vi "test_delay.vi"() -> ()   [LabVIEW 2013]
uses:
  <vilib>/rvi/FXPMathLib/FxpConvert/subVIs/nifxpmath_Convert_SimConfig.ctl
  <vilib>/fxp/LVFixedPointQuantizationPolicyTypeDef.ctl
  <vilib>/fxp/LVFixedPointOverflowPolicyTypeDef.ctl
  <vilib>/rvi/FXPMathLib/FxpConvert/simVIs/DllFxpConvertTemp_sub.vi
  <vilib>/rvi/FXPMathLib/FxpConvert/XNode/nifxpmath_Convert.xnode
  <vilib>/rvi/FXPMathLib/FxpMul/XNode/nifxpmath_Multiplier.xnode
  <vilib>/rvi/FXPMathLib/sim/FxpSim.dll
panel:
  out "Array 2":fxp<+/-,32,16>[](array[numeric])
  out "Array":fxp<+/-,16,14>[](array[numeric])
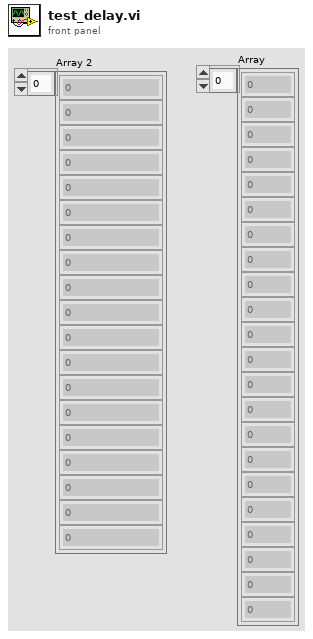
[diagram p1: front panel]
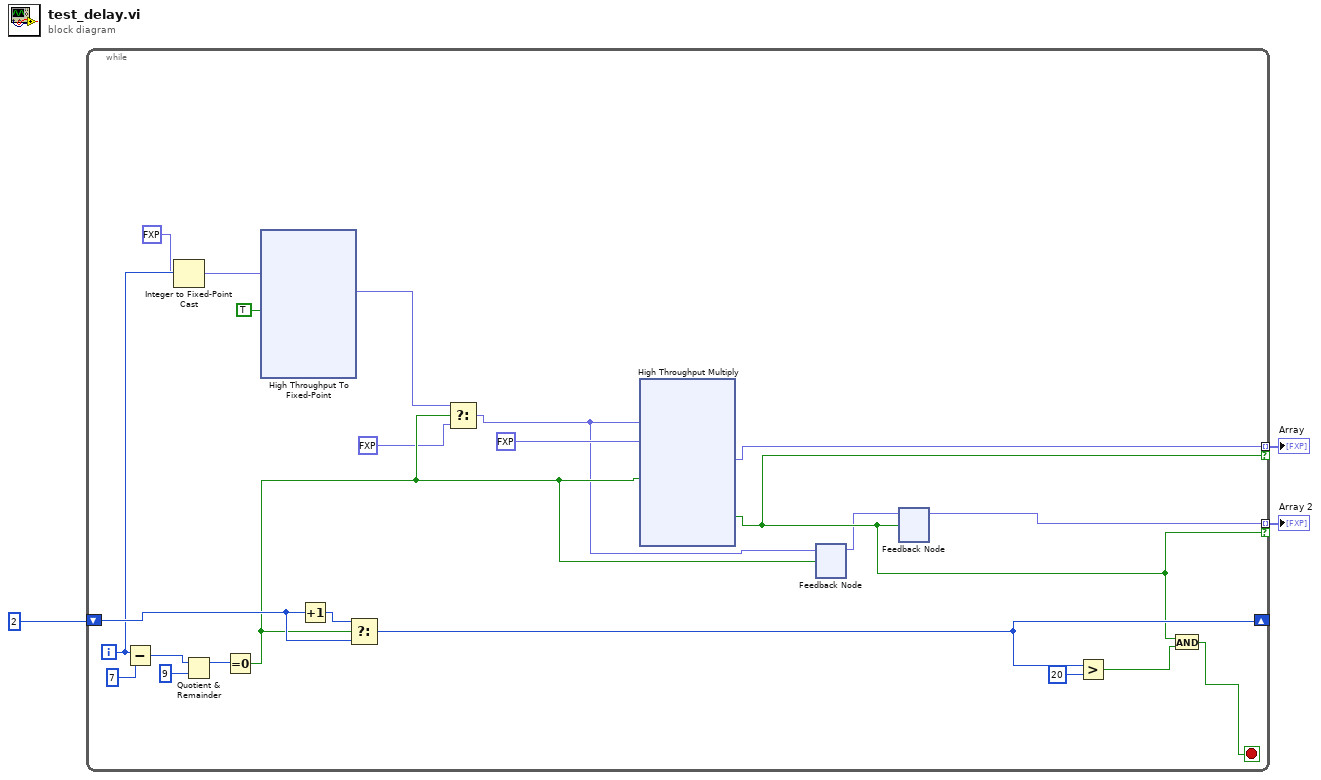
[diagram p0: block diagram]
diagram:
  n1 = while {
    shift-right: [w17] -> _
    shift-left: 2 ("y") -> [w23]
    tunnel: [w4] -> w1 mode=indexing if=w14
    tunnel: [w15] -> w2 mode=indexing if=w14
    i -> [w10]
    stop <- w19 stop-if-true
    n2 = Subtract(x=w10, y=7) -> (x-y=w21:i32)
    n3 = Integer to Fixed-Point Cast(fixed-point type=fxp<+/-,32,32> 0.0, integer=w10) -> (fixed-point=w8:fxp<+/-,32,32>)
    n4 = Quotient & Remainder(x=w21, y=9) -> (x-y*floor(x/y)=w25:i32)  [unwired: 1 out]
    n5 = Equal To 0?(x=w25) -> (x = 0?=w13:bool)
    n6 = xnode "High Throughput To Fixed-Point"("x"=w8, "input valid"=TRUE) -> ("y"=w7:fxp<+/-,32,16>)  [unwired: 1 in, 2 out]
    n7 = Increment(x=w23) -> (x+1=w24:i32)
    n8 = Select(t=w24, s=w13, f=w23) -> (s? t:f=w17:i32)
    n9 = Select(t=w7, s=w13, f=fxp<+/-,32,16> 0.0 ("x")) -> (s? t:f=w11:fxp<+/-,32,16>)
    n10 = xnode ("High Throughput Multiply")("x"=w11, "y"=fxp<+/-,32,16> 5.0 ("x"), "input valid"=w13) -> ("x*y"=w15:fxp<+/-,16,14>, "output valid"=w14:bool)  [unwired: 1 in, 1 out]
    n11 = feedback #1() -> (w5:fxp<+/-,32,16>)  [unwired: 1 in]
    n12 = feedback-in #1(w11, w13) -> ()
    n13 = feedback #2() -> (w4:fxp<+/-,32,16>)  [unwired: 1 in]
    n14 = feedback-in #2(w5, w14) -> ()
    n15 = Greater?(x=w17, y=20) -> (0:w20:bool)
    n16 = And(x=w14, y=w20) -> (x .and. y?=w19:bool)
  }
  "Array" <- w2
  "Array 2" <- w1
